vi "add_line_enface.vi"(6 "Output Line":i32, 9 "Out Image":dbl[][](array[numeric]), 10 "Input Line":dbl=74.0, 11 "Image":T1) -> (2 "Out Image":dbl[][](array[numeric]))   [LabVIEW 2016]
uses:
  <vilib>/vision/Image Controls.llb/IMAQ Image.ctl
  <vilib>/vision/NI_Vision_Development_Module.lvlib
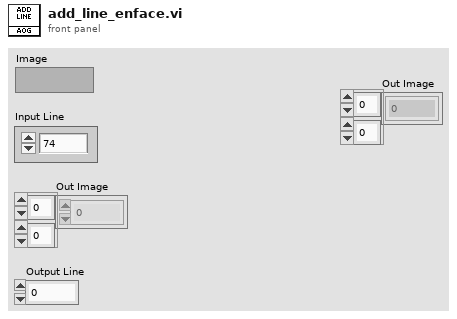
[diagram p1: front panel]
types:
  T1 = typedef "IMAQ Image.ctl" = refnum<image>
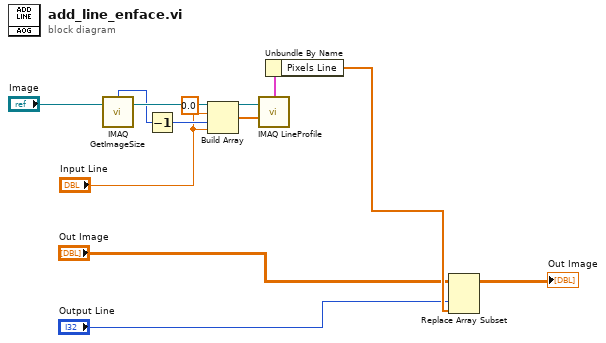
[diagram p0: block diagram]
diagram:
  n1 = call "IMAQ GetImageSize"("Image"="Image") -> ("X Resolution"=w7:i32)  [unwired: 3 in, 2 out]
  n2 = Decrement(x=w7) -> (x-1=w6:i32)
  n3 = Build Array(0.0 ("element"), "Input Line", w6, "Input Line") -> (w9:dbl[])
  n4 = call "IMAQ LineProfile"("Line Coordinates"=w9, "Image"="Image") -> ("Line Graph"=w4:cluster{"x0":sgl, "dx":sgl, "Pixels Line":sgl[]})  [unwired: 3 in, 3 out]
  n5 = Unbundle By Name(w4) -> ("Pixels Line"=w10:sgl[])
  n6 = Replace Array Subset(array="Out Image", new element=w10, index (col)="Output Line") -> (→"Out Image":dbl[][])  [unwired: 1 in]
